vi "Active Transfer Groups.vi"(8 "error in (no error)":errorcluster, 11 "Plugin in":refnum<class "Plugin.lvclass">) -> (0 "error out":errorcluster, 3 "Plugin out":refnum<class "Plugin.lvclass">)   [LabVIEW 2017, in "DSF Core.lvlib" / "Plugin.lvclass"]
uses:
  Plugin.lvclass
  Plugin.lvclass/Plugin.ctl
  Timing/Timing.lvclass/Timing.ctl
  Transfer Group/Transfer Group.lvclass/Transfer Group.ctl
  Transfer Group/Get Timing.vi
  Timing/Is Active Cycle.vi
  Get Timing.vi
  Timing/Get Iteration.vi
  Timing/Get Decimation.vi
  Timing/Get Offset.vi
  Transfer Group/Transfer Group.lvclass
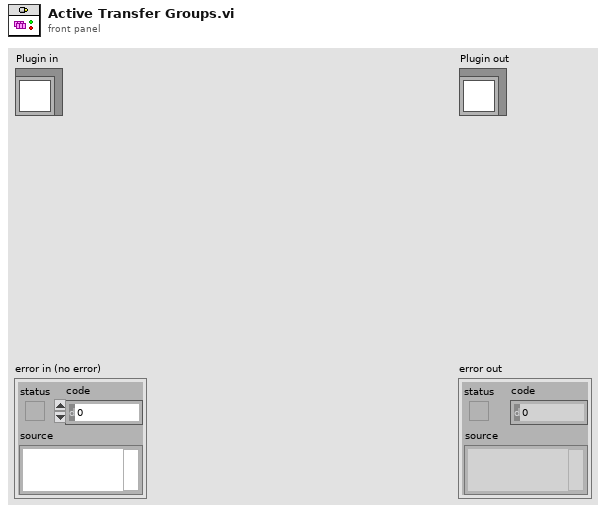
[diagram p1: front panel]
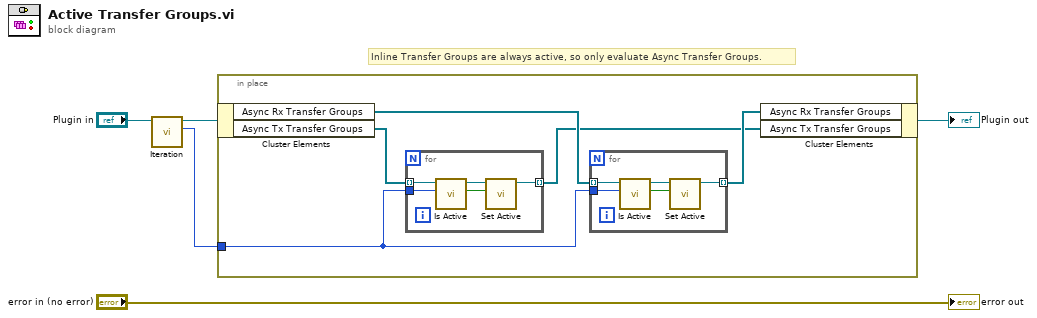
[diagram p0: block diagram]
diagram:
  # "Inline Transfer Groups are always active, so only evaluate Async Transfer Groups."
  n1 = call "Iteration.vi"("Plugin in"="Plugin in") -> ("Iteration"=w2:u64, "Plugin out"=w3:refnum<class "Plugin.lvclass">)  [unwired: 9 in]
  n2 = in-place {
    in-place-border: w2 -> [w6]
    n3 = in-place-cluster #1(w3) -> ("Async Rx Transfer Groups"=w8:refnum<class "Transfer Group.lvclass">[], "Async Tx Transfer Groups"=w10:refnum<class "Transfer Group.lvclass">[])
    n4 = for {
      tunnel: w10 -> [w20] mode=indexing
      tunnel: [w17] -> w7 mode=indexing
      tunnel: w6 -> [w16]
      n5 = call "Is Active.vi"("cycle count"=w16, "Transfer Group in"=w20) -> ("active this cycle?"=w18:bool, "Transfer Group out"=w19:refnum<class "Transfer Group.lvclass">)  [unwired: 8 in]
      n6 = call "Set Active.vi"("active"=w18, "Transfer Group in"=w19) -> ("Transfer Group out"=w17:refnum<class "Transfer Group.lvclass">)  [unwired: 9 in]
    }
    n7 = for {
      tunnel: w8 -> [w15] mode=indexing
      tunnel: [w12] -> w9 mode=indexing
      tunnel: w6 -> [w11]
      n8 = call "Is Active.vi"("cycle count"=w11, "Transfer Group in"=w15) -> ("active this cycle?"=w13:bool, "Transfer Group out"=w14:refnum<class "Transfer Group.lvclass">)  [unwired: 8 in]
      n9 = call "Set Active.vi"("active"=w13, "Transfer Group in"=w14) -> ("Transfer Group out"=w12:refnum<class "Transfer Group.lvclass">)  [unwired: 9 in]
    }
    n10 = in-place-cluster #1("Async Rx Transfer Groups"=w9, "Async Tx Transfer Groups"=w7) -> (→"Plugin out":refnum<class "Plugin.lvclass">)
  }
  "error out" <- "error in (no error)"
